vi "Module ID.vi"(11 "System Config Module in":refnum<class "System Config Module.lvclass">) -> (2 "Module ID":string)   [LabVIEW 2020, in "Volatus.lvlib" / "System Config Module.lvclass"]
uses:
  System Config Module.lvclass
  System Config Module.lvclass/System Config Module.ctl
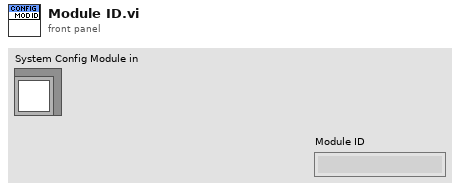
[diagram p1: front panel]
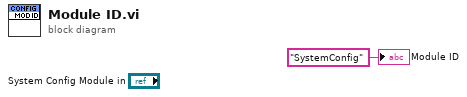
[diagram p0: block diagram]
diagram:
  "Module ID" <- "SystemConfig" ("Module ID")
